vi "AprilTag Target Package Code 1 with integrated camera.vi"(1 "Instance":i32) -> (0 "Camera Name":string="cam0")   [LabVIEW 2025]
uses:
  <vilib>/vision/Image Controls.llb/IMAQ Image.ctl
  <vilib>/Utility/config.llb/NI_LVConfig.lvlib
  Camera Set Up/Event/Event Setup Types.ctl
  State Machine/AprialTag States.ctl
  State Machine/AprialTag Main Cluster.ctl
  Steam Type.ctl
  <vilib>/ptbypt/NI_PtbyPt.lvlib
  <vilib>/Utility/config.llb/Read Key (String).vi
  <vilib>/Utility/config.llb/Write Key (String).vi
  Camera Set Up/Ctrl/White Balance.ctl
  <vilib>/userDefined/High Color/IMAQdx.ctl
  Main State Machine/Ctrl's/Main States.ctl
  Main State Machine/Ctrl's/Main Queue.ctl
  Main State Machine/Ctrl's/Main Cluster.ctl
  <vilib>/vision/driver/NI_Vision_Acquisition_Software.lvlib
  <vilib>/vision/NI_Vision_Development_Module.lvlib
  <resource>/objmgr/imaqdx.rc
  <vilib>/regexp/Match Regular Expression.xnode
  cef373c4-9c7f-4541-9f08-8c9f27cfdef0.vi
  Camera Info.ctl
panel:
  in  "Main":enum32{"Page 1", "Page 2", "Page 3"}(tab)
  out "Target Pitch":dbl[](array[numeric]) caption="Tag Pitch (deg)" format="%.1f"
  out "Target Yaw":dbl[](array[numeric]) caption="Tag Yaw (deg)" format="%.1f"
  out "Tag ID":dbl[](array[numeric]) caption="Tag Number"
  out "Image":T1(plugin-control)
  in  "Settings":bool
  in  "Save":bool
  in  "Tools":bool
  out "FPS":dbl format="%#.0f"
  out "Distance":dbl[](array[numeric]) caption="Tag Distance (in)" format="%.1f"
  out "Angle":dbl[](array[numeric]) caption="Center Angle (deg)" format="%.1f"
  out "Height":i32=360
  out "Width":i32=640
  in  "Home":bool
  in  "Robot Calibration Cluster":T2={"Camera Height on robot (in)"=9.5, "Camera Angle on the robot (deg)"=2.5, "Camera FOV Vert View Angle (deg)"=26.5, "Camera FOV Hor View Angle (deg)"=68.5, "Camera Focal Length (mm)"=10.0, "Target size (in)"=6.5} {"Camera FOV Hor View Angle (deg)" format="%#_13g"; "Camera Focal Length (mm)" format="%#_13g"; "Target size (in)" format="%#_13g"; "Camera FOV Vert View Angle (deg)" format="%#_13g"; "Camera Angle on the robot (deg)" format="%#_13g"; "Camera Height on robot (in)" format="%#_13g"}
  in  "decimate":dbl=4.0 format="%#_13g"
  out "Data to Send":dbl[][](array[numeric])
  out "Greyscale":bool
  out "Height 2":u32=360
  out "Width 2":u32=640
  out "Frames per Second":dbl format="%#.1f"
  in  "Gamma":i32(slide)=50 min=1 max=100 scale=0.0..100.0
  in  "Brightness":i32(slide)=50 min=1 max=100 scale=0.0..100.0
  in  "Exposure":i32(slide)=50 min=1 max=100 scale=0.0..100.0
  in  "Save 2":bool caption="Save"
  in  "Close":bool
  in  "Gain":i32(slide)=50 min=1 max=100 scale=0.0..100.0
  in  "Contrast":i32(slide)=50 min=1 max=100 scale=0.0..100.0
  in  "Sharpness":i32(slide)=50 min=1 max=100 scale=0.0..100.0
  in  "VideoMode":u16(ring)=20 items=["640x480 MJPG 60.00fps", "640x480 YUY2 60.00fps", "1280x720 MJPG 60.00fps", "1280x720 YUY2 60.00fps", "1600x1304 MJPG 60.00fps", "1600x1304 YUY2 60.00fps"]
  in  "White Balance":T3=enum."Hold current"
  out "Camera Name 2":string="cam1"
  out "Camera Image":T1(plugin-control)
  in  "Hue":i32(slide)=50 min=1 max=100 scale=0.0..100.0
  in  "Saturation":i32(slide)=50 min=1 max=100 scale=0.0..100.0
  out "Camera Name 3":string="cam0"
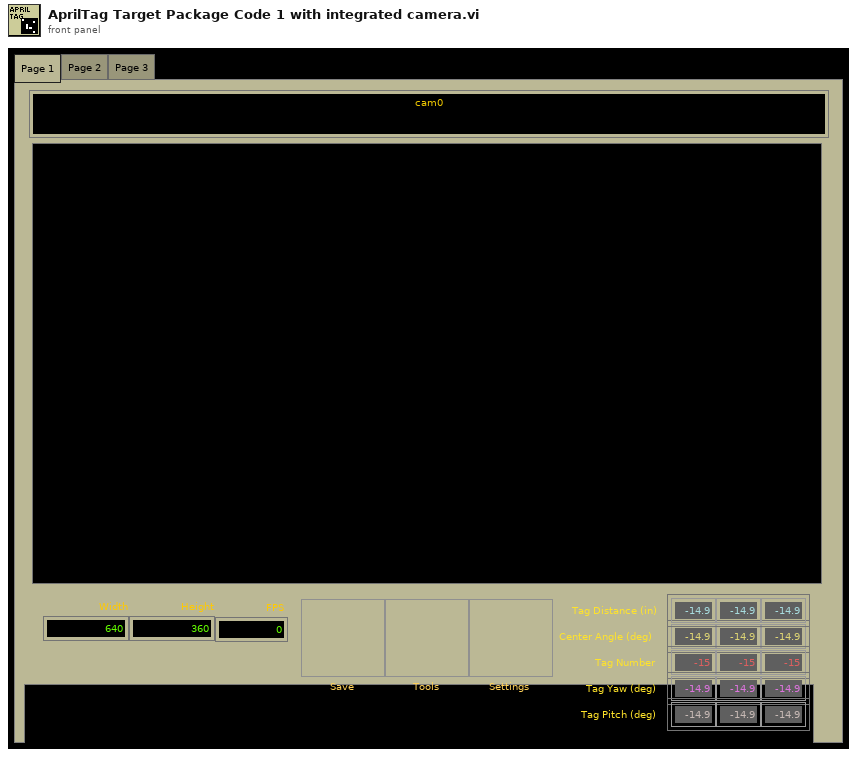
[diagram p1: front panel]
types:
  T1 = typedef "IMAQ Image.ctl" = refnum<image>
  T2 = typedef "Camera Info.ctl" = cluster{"Camera Height on robot (in)":dbl, "Camera Angle on the robot (deg)":dbl, "Camera FOV Vert View Angle (deg)":dbl, "Camera FOV Hor View Angle (deg)":dbl, "Camera Focal Length (mm)":dbl, "Target size (in)":dbl}
  T3 = typedef "White Balance.ctl" = enum16{"Auto", "Fixed indoor", "Fixed outdoor 1", "Fixed outdoor 2", "Fixed fluorescent 1", "Fixed fluorescent 2", "Hold current", "Custom"}
  T4 = typedef "AprialTag Main Cluster.ctl" = cluster{"AprilTage FIFO":T5[], "Camera Name":string, "AprilTag path":path, "Control Ref's":refnum<vi>[], "Main Image":T1, "Timeout":i32, "EDIT Settings":bool, "Calibration path":path, "Camera Number":dbl}
  T5 = typedef "AprialTag States.ctl" = enum16{"Message Dispatcher", "INI", "Open", "Save", "Exit"}
  T6 = typedef "Main Cluster.ctl" = cluster{"Main Queue":T7, "error":errorcluster, "Camera":T9, "Camera Session":T9, "Image In":T1, "White Balance":T3, "Attr String":string[], "Values":u16[], "VideoMode":u16, "Exposure":i32, "Reset":bool, "Greyscale":bool, "Controls":refnum<vi>[], "INI path":path, "INI File Found":bool, "Open And Save Controls":refnum<vi>[]}
  T7 = typedef "Main Queue.ctl" = T8[]
  T8 = typedef "Main States.ctl" = enum16{"Message Dispatcher", "INI", "End Session", "Camera Process Settings", "Get Values", "Get VideoMode", "Open Settings", "Save Settings", "Set Value", "Set VideoMode", "Set WB", "Setup Camera", "Start Session", "Exit"}
  T9 = typedef "IMAQdx.ctl" = refnum<k21>
  T10 = typedef "Event Setup Types.ctl" = enum16{"Default", "Camera Loop Started", "GreyScale", "Reset Team Number", "Save Data", "Exit"}
  T11 = enum32{"Invalid", "Standard", "Closed", "Hidden", "Minimized", "Maximized"}
  T12 = enum32{"Invalid", "Default", "Floating", "Floating/Auto-Hide", "Modal"}
  T13 = typedef "Steam Type.ctl" = enum8{"Unknown", "Apriltag", "Algae", "Coral"}
  T14 = typedef "Event Setup Types.ctl" = enum16{"Default", "Camera Loop Started", "Close Settings", "GreyScale", "Open Front Panel", "Reset Team Number", "Save Data", "Exit"}
  T15 = cluster{"tag ID":i32, "Center":cluster{"X":dbl, "Y":dbl}, "homography matrix":dbl[], "decision margin":dbl, "Hamming Dist":i32, "corner points":cluster{"X":dbl, "Y":dbl}[], "Tag Family":string}[]
  T16 = typedef "AprilTag Target Fields.ctl" = cluster{"diameter points":cluster{"first point":cluster{"x":dbl, "y":dbl}, "projected point":cluster{"x":dbl, "y":dbl}}, "normalized center":cluster{"x":dbl, "y":dbl}, "Overall Score":dbl, "Distance (ft)":dbl, "Offset Angle":dbl, "Tag corner points":cluster{"X":dbl, "Y":dbl}[], "Tag Center":cluster{"X":dbl, "Y":dbl}, "Tag Yaw":dbl, "Tag Pitch":dbl, "Target Roll (deg)":dbl, "AprilTag Number":i32, "homography matrix":dbl[]}
  T17 = typedef "Image Type" = u32
  T18 = typedef "NI_LVConfig.lvlib/Config Data RefNum.ctl" = refnum<k1>
  T19 = cluster{"Video Mode":u32, "Video Mode Name":string}[]
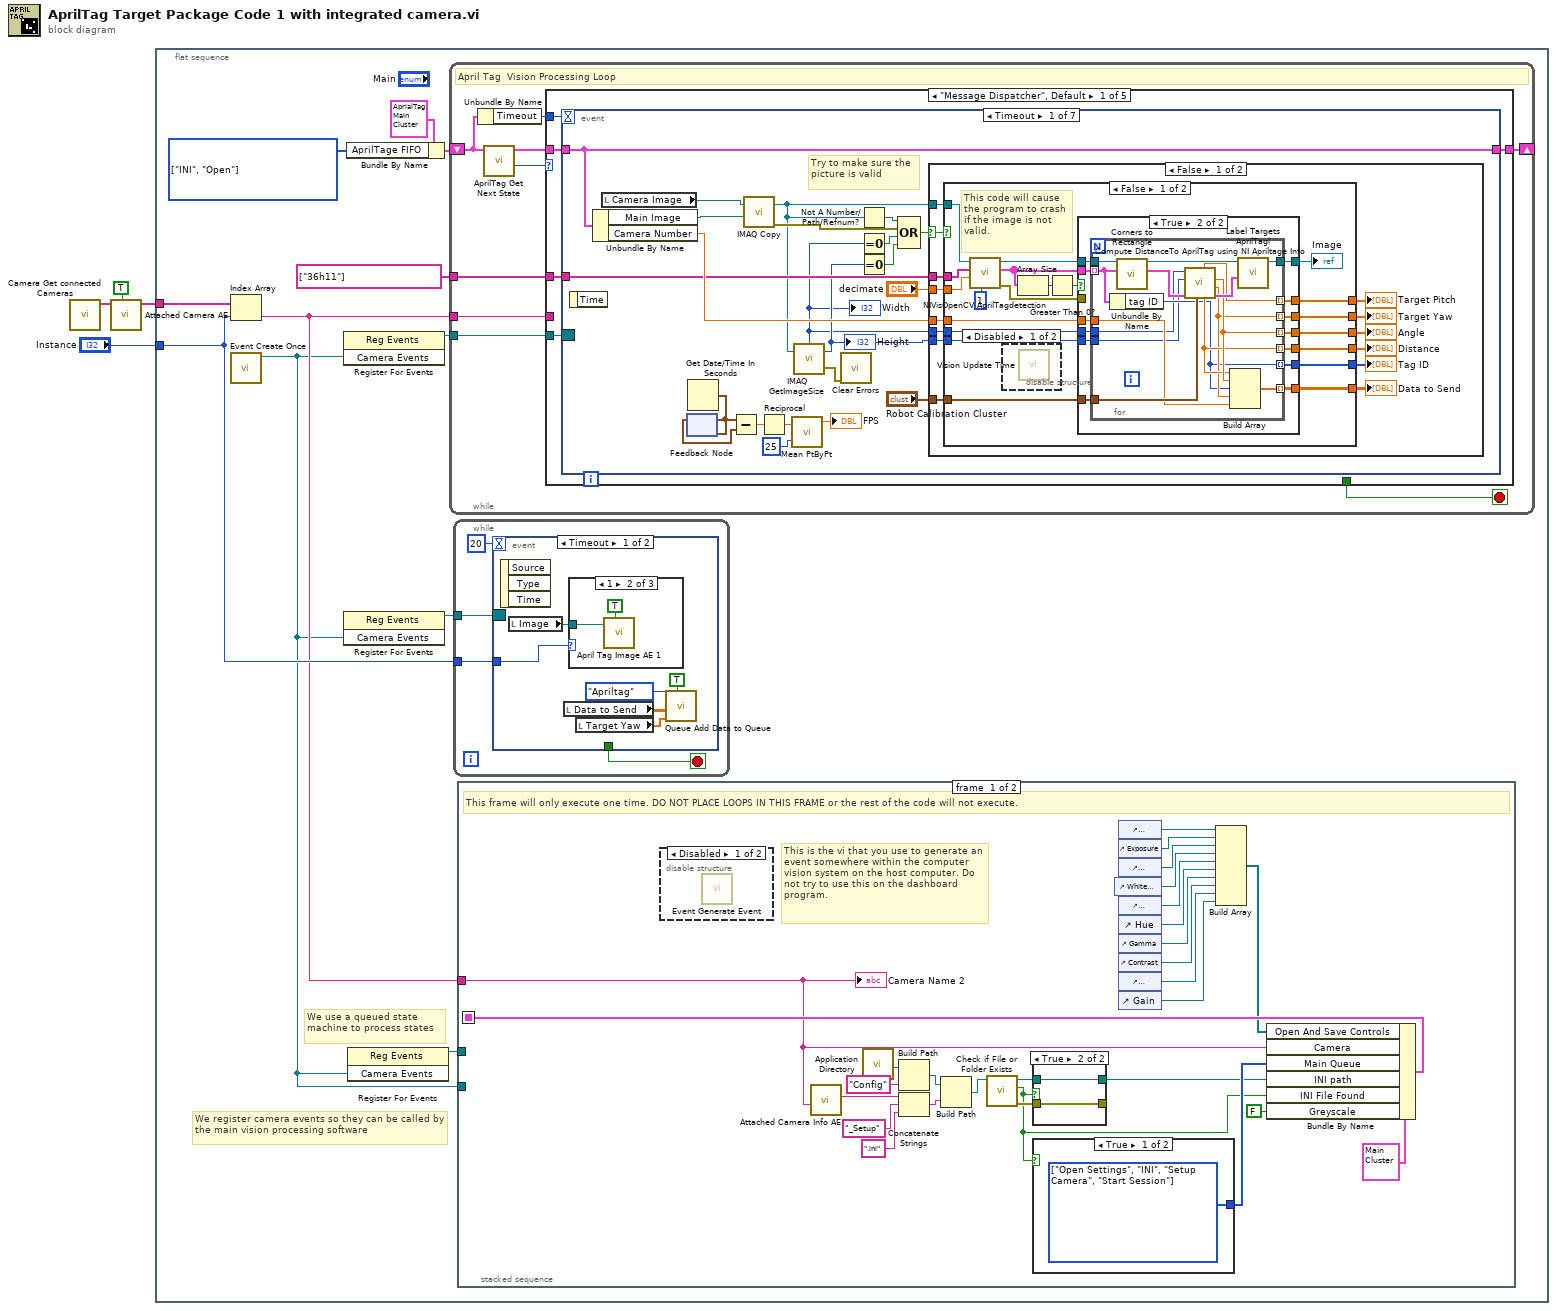
[diagram p0: block diagram]
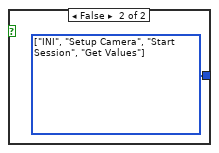
[diagram p2: hidden frame]
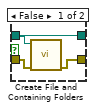
[diagram p3: hidden frame]
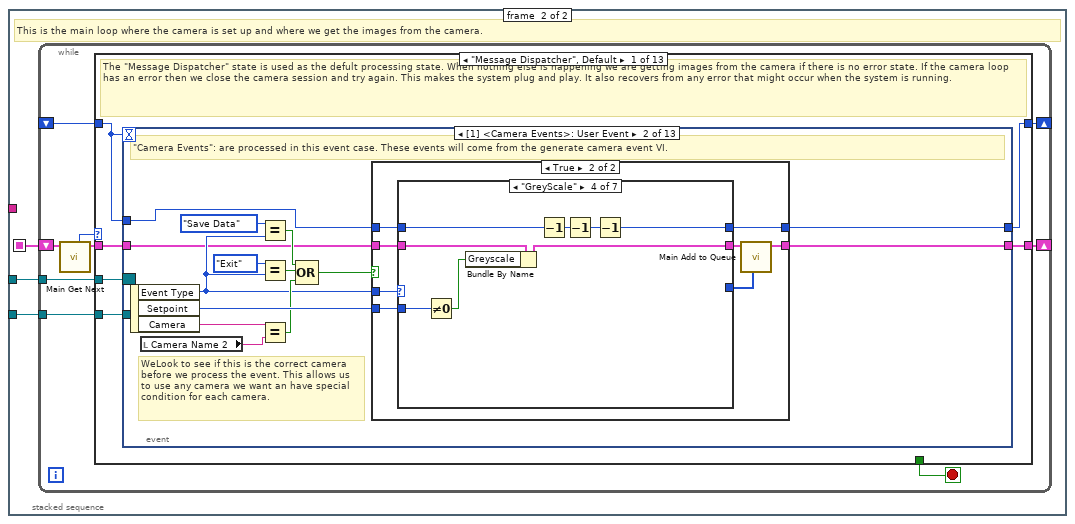
[diagram p5: hidden frame]
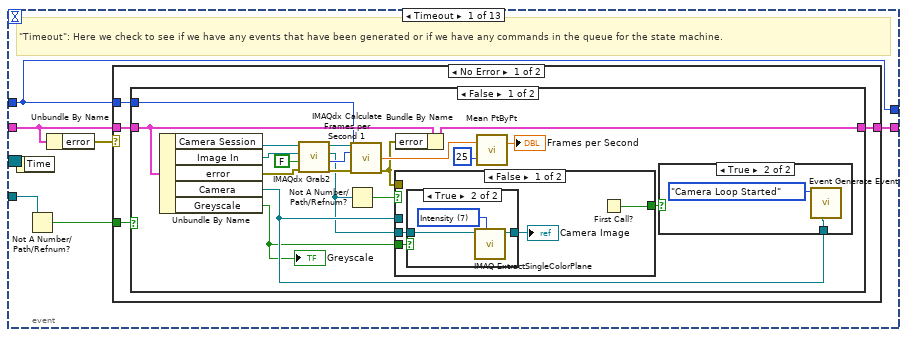
[diagram p6: hidden frame]
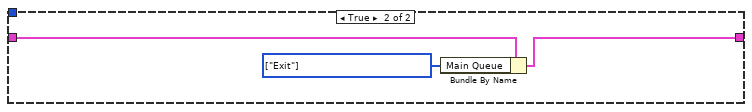
[diagram p10: hidden frame]
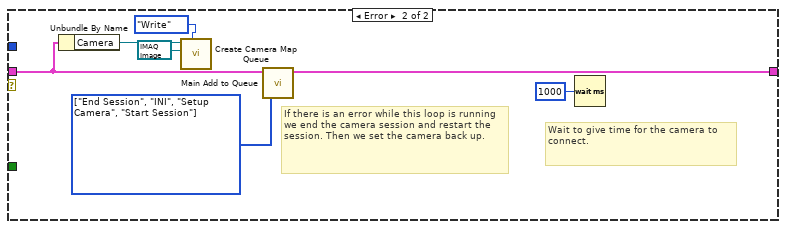
[diagram p11: hidden frame]
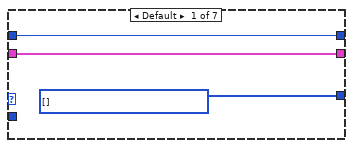
[diagram p13: hidden frame]
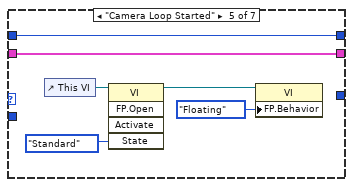
[diagram p16: hidden frame]
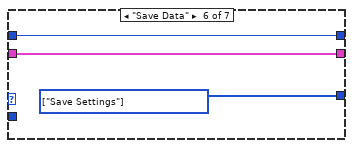
[diagram p17: hidden frame]
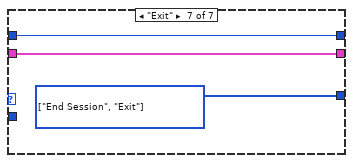
[diagram p18: hidden frame]
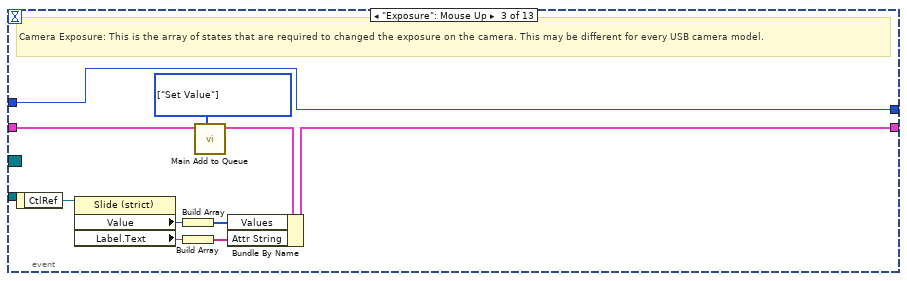
[diagram p19: hidden frame]
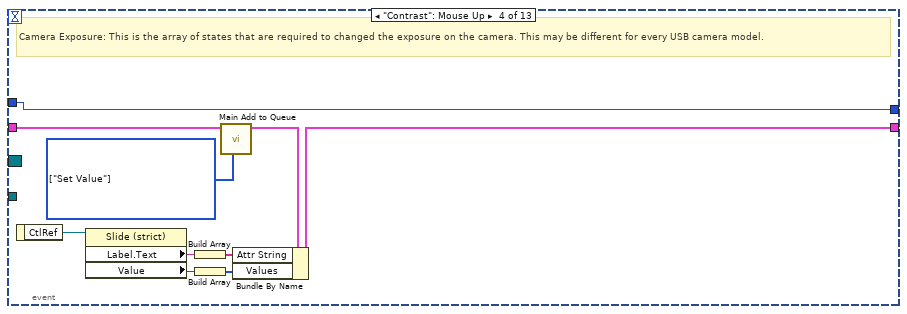
[diagram p20: hidden frame]
diagram:
  n1 = call "Camera Get connected Cameras.vi"() -> ("Camera List"=w4:string[])  [unwired: 10 in, 1 out]
  n2 = call "Attached Camera AE.vi"("Update"=TRUE, "Camera List in"=w4) -> ("Camera List out"=w2:string[])  [unwired: 9 in]
  n3 = flat-sequence {
    tunnel: w2 -> [w8]
    tunnel: "Instance" -> [w7]
    frame #0 {
      w12 = T5[] [enum."INI", enum."Open"] items=["Message Dispatcher", "INI", "Open", "Save", "Exit"] ("AprilTage FIFO")
      # "We register camera events so they can be called by the main vision processing software"
      # "We use a queued state machine to process states"
      n4 = Index Array(array=w8, index=w7) -> (element=w6:string)
      n5 = call "Event Create Once.vi"() -> ("Camera Events"=w5:refnum<user-event>)  [unwired: 10 in, 1 out]
      n6 = register-events(w5) -> (reference out=w15:refnum<event-registration>)  [unwired: 2 in, 1 out]
      n7 = register-events(w5) -> (reference out=w10:refnum<event-registration>)  [unwired: 2 in, 1 out]
      n8 = Bundle By Name(cluster=T4 {"AprilTage FIFO"=[], "Camera Name"="", "AprilTag path"=path "", "Control Ref's"=[], "Main Image"=refnum, "Timeout"=5, "EDIT Settings"=FALSE, "Calibration path"=path "", "Camera Number"=0.0} ("AprilTag Main Cluster out"), "AprilTage FIFO"=w12) -> (w13:T4)
      n9 = register-events(w5) -> (reference out=w9:refnum<event-registration>)  [unwired: 2 in, 1 out]
      n10 = while {
        tunnel: w15 -> [w762]
        shift-right: [w758] -> _
        shift-left: w13 -> [w756]
        tunnel: string[] ["36h11"] ("Tag Familys") -> [w755]
        tunnel: w6 -> [w754]
        stop <- w761 stop-if-true
        # "April Tag  Vision Processing Loop"
        n11 = Unbundle By Name(w756) -> ("Timeout"=w757:i32)
        n12 = call "AprilTag Get Next State.vi"("AprilTag Main Cluster in"=w756) -> ("Next State"=w759:T5, "AprilTag Main Cluster out"=w760:T4)  [unwired: 9 in]
        n13 = case shown="\"Message Dispatcher\", Default" w759 {
          tunnel: w762 -> [w767 _ _ _ _]
          tunnel: [_ _ _ _ TRUE] -> w761
          tunnel: w760 -> [w765 w914 w931 w968 w984]
          tunnel: [w766 w913 w930 w968 w984] -> w758
          tunnel: w757 -> [w764 _ _ _ _]
          tunnel: w755 -> [w763 _ _ _ _]
          tunnel: w754 -> [_ w890 w920 _ _]
          frame "Message Dispatcher", Default {
            n14 = event shown="[0] Timeout" {
              selector: w767 -> [_ _ _ _ _ _ _]
              dyn-events: _ -> [_ _ _ _ _ _ _]
              timeout: w764 -> [_ _ _ _ _ _ _]
              tunnel: w765 -> [w789 w856 w879 w880 w882 w886 w888]
              tunnel: [w789 w858 w878 w880 w882 w885 w888] -> w766
              tunnel: w763 -> [w785 _ _ _ _ _ _]
              event Timeout {
                # "Try to make sure the picture is valid"
                n15 = event-data() -> ()  [unwired: 1 in, 1 out]
                n16 = Unbundle By Name(w789) -> ("Main Image"=w784:T1, "Camera Number"=w787:dbl)
                n17 = local read "Camera Image"() -> (w768:T1)
                n18 = Get Date/Time In Seconds() -> (seconds since 1Jan1904=w773:timestamp)
                n19 = feedback #1(w773) -> (w774:timestamp)
                n20 = feedback-in #1(w773) -> ()
                n21 = Subtract(x=w773, y=w774) -> (x-y=w771:dbl)
                n22 = call "IMAQ Copy"("Image Dst"=w784, "Image Src"=w768) -> ("error out"=w783:errorcluster, "Image Dst Out"=w776:T1)  [unwired: 4 in]
                n23 = Reciprocal(x=w771) -> (1/x=w772:dbl)
                n24 = call <vilib>:"Mean PtByPt.vi"("x"=w772, "sample length"=25) -> ("mean"=→"FPS":dbl)  [unwired: 2 in, 1 out]
                n25 = call "IMAQ GetImageSize"("Image"=w776) -> ("Y Resolution"=w778:i32, "X Resolution"=w777:i32, "error out"=w775:errorcluster)  [unwired: 3 in]
                "Height" <- w778
                "Width" <- w777
                n26 = call <vilib>:"Clear Errors.vi"("error in (no error)"=w775) -> ()  [unwired: 5 in, 2 out]
                n27 = Not A Number/Path/Refnum?(number/path/refnum=w776) -> (NaN/Path/Refnum?=w782:bool)
                n28 = Equal To 0?(x=w777) -> (x = 0?=w780:bool)
                n29 = Equal To 0?(x=w778) -> (x = 0?=w779:bool)
                n30 = Compound Arithmetic op=OR(w782, w783, w780, w779) -> (w781:bool)
                n31 = case shown="False" w781 {
                  selector: w781 -> [w794 _]
                  tunnel: w785 -> [w803 _]
                  tunnel: "Robot Calibration Cluster" -> [w802 _]
                  tunnel: w787 -> [w797 _]
                  tunnel: w776 -> [w796 _]
                  tunnel: "decimate" -> [w795 _]
                  tunnel: w778 -> [w792 _]
                  tunnel: w777 -> [w791 _]
                  frame False {
                    n32 = case shown="False" w794 {
                      tunnel: w803 -> [w823 _]
                      tunnel: w802 -> [w822 _]
                      tunnel: [w817 _] -> w790
                      tunnel: [w816 _] -> w801
                      tunnel: [w815 _] -> w793
                      tunnel: [w814 _] -> w800
                      tunnel: [w813 _] -> w799
                      tunnel: [w812 _] -> w798
                      tunnel: w797 -> [w811 _]
                      tunnel: w796 -> [w808 _]
                      tunnel: w795 -> [w809 _]
                      tunnel: w792 -> [w805 _]
                      tunnel: w791 -> [w804 _]
                      frame False {
                        # "This code will cause the program to crash if the image is not valid."
                        n33 = call "NIVisOpenCV AprilTagdetection.vi"("threads"=1, "decimate"=w809, "Tag Familys"=w823, "Image Src"=w808) -> ("error out"=w818:errorcluster, "Detected Tags"=w821:T15, "Image Dst Out"=w807:T1)  [unwired: 4 in, 1 out]
                        n34 = disable-structure shown="Disabled" {
                          frame Disabled {
                            n35 = call "Vision Update Time.vi"() -> ()  [unwired: 12 in]
                          }
                          frame Enabled {
                          }
                        }
                        n36 = Array Size(array=w821) -> (size(s)=w820:i32)
                        n37 = Greater Than 0?(x=w820) -> (x > 0?=w819:bool)
                        n38 = case shown="True" w819 {
                          tunnel: w807 -> [w824 w837]
                          tunnel: w821 -> [_ w836]
                          tunnel: [w824 w827] -> w810
                          tunnel: w818 -> [_ _]
                          tunnel: w822 -> [_ w835]
                          tunnel: [_ w834] -> w817
                          tunnel: [_ w833] -> w816
                          tunnel: [_ w832] -> w815
                          tunnel: [_ w831] -> w814
                          tunnel: [_ w830] -> w813
                          tunnel: [_ w829] -> w812
                          tunnel: w811 -> [_ w828]
                          tunnel: w805 -> [_ w826]
                          tunnel: w804 -> [_ w825]
                          frame False {
                          }
                          frame True {
                            n39 = for {
                              tunnel: w836 -> [w851] mode=indexing
                              tunnel: w837 -> [w840]
                              tunnel: [w852] -> w827
                              tunnel: [w841] -> w831 mode=indexing
                              tunnel: [w846] -> w829 mode=indexing
                              tunnel: [w848] -> w830 mode=indexing
                              tunnel: w835 -> [w847]
                              tunnel: [w845] -> w832 mode=indexing
                              tunnel: [w844] -> w834 mode=indexing
                              tunnel: [w843] -> w833 mode=indexing
                              tunnel: w828 -> [w842]
                              tunnel: w826 -> [w839]
                              tunnel: w825 -> [w838]
                              n40 = Unbundle By Name(w851) -> ("tag ID"=w841:i32)
                              n41 = call "Corners to Rectangle.vi"("tag info"=w851) -> ("output cluster"=w850:T16)  [unwired: 10 in]
                              n42 = call "Compute DistanceTo AprilTag using NI Apriltage Info.vi"("Robot Calibration Cluster"=w847, "results"=w850, "Y Resolution"=w839, "X Resolution"=w838) -> ("results out"=w849:T16, "Target Yaw (deg)"=w845:dbl, "Offset Angle"=w848:dbl, "Distance from target (in)"=w846:dbl, "Target Pitch (deg)"=w843:dbl)  [unwired: 2 in, 1 out]
                              n43 = Build Array(w846, w848, w841, w845, w842) -> (w844:dbl[])
                              n44 = call "Label Targets AprilTagl.vi"("results"=w849, "Image in"=w840) -> ("Image out"=w852:T1)  [unwired: 9 in]
                            }
                          }
                        }
                        "Image" <- w810
                      }
                      frame True {
                      }
                    }
                    "Distance" <- w798
                    "Angle" <- w799
                    "Tag ID" <- w800
                    "Target Yaw" <- w793
                    "Target Pitch" <- w801
                    "Data to Send" <- w790
                  }
                  frame True {
                  }
                }
              }
              event User Event {
                n45 = event-data() -> ("Camera"=w854:string, "Event Type"=w857:T10)  [unwired: 1 in]
                n46 = Unbundle By Name(w856) -> ("Camera Name"=w855:string)
                n47 = Equal?(x=w855, y=w854) -> (x = y?=w853:bool)
                n48 = case shown="\"Save Data\"" w857 {
                  tunnel: w856 -> [w859 w861 w866 w867 w868 w869 w872 w875]
                  tunnel: [w859 w865 w866 w867 w868 w869 w871 w874] -> w858
                  tunnel: w853 -> [_ _ _ _ _ _ _ _]
                  frame "Default" {
                  }
                  frame "Camera Loop Started" {
                    n49 = Unbundle By Name(w861) -> ("Camera Name"=w860:string)
                    n50 = call "Event Generate Event.vi"("Camera Name"=w860, "Setpoint"=i64 1, "Event Type"=Event_Setup_Types."GreyScale") -> ()  [unwired: 9 in]
                    n51 = Bundle By Name(cluster=w861, "Timeout"=10) -> (w865:T4)
                  }
                  frame "Default" {
                  }
                  frame "GreyScale" {
                  }
                  frame "Camera Loop Started" {
                  }
                  frame "Reset Team Number" {
                  }
                  frame "Save Data" {
                    w870 = T5[] [enum."Save"] items=["Message Dispatcher", "INI", "Open", "Save", "Exit"] ("AprilTage FIFO")
                    n52 = Bundle By Name(cluster=w872, "AprilTage FIFO"=w870) -> (w871:T4)
                  }
                  frame "Exit" {
                    w873 = T5[] [enum."Exit"] items=["Message Dispatcher", "INI", "Open", "Save", "Exit"] ("AprilTage FIFO")
                    n53 = Bundle By Name(cluster=w875, "AprilTage FIFO"=w873) -> (w874:T4)
                  }
                }
              }
              event "Camera Name": Value Change {
                w877 = T5[] [enum."INI", enum."Save"] items=["Message Dispatcher", "INI", "Open", "Save", "Exit"] ("AprilTage FIFO")
                n54 = event-data() -> ("NewVal"=w876:string)  [unwired: 1 in]
                n55 = Bundle By Name(cluster=w879, "Camera Name"=w876, "AprilTage FIFO"=w877) -> (w878:T4)
              }
              event "Tools": Mouse Up {
                n56 = event-data() -> ()  [unwired: 1 in, 1 out]
                n57 = property on="Main" class="TabCtl (strict)"("Value"=enum32{"Page 1", "Page 2"}."Page 2" ("Main")) -> ()  [unwired: 2 in, 2 out]
              }
              event "Home": Mouse Up {
                n58 = event-data() -> ()  [unwired: 1 in, 1 out]
                n59 = property on="Main" class="TabCtl (strict)"("Value"=enum32{"Page 1", "Page 2"}."Page 1" ("Main")) -> ()  [unwired: 2 in, 2 out]
              }
              event "Save": Mouse Up {
                w884 = T5[] [enum."Save"] items=["Message Dispatcher", "INI", "Open", "Save", "Exit"] ("AprilTage FIFO")
                n60 = event-data() -> ()  [unwired: 1 in, 1 out]
                n61 = Bundle By Name(cluster=w886, "AprilTage FIFO"=w884) -> (w885:T4)
              }
              event "Settings": Mouse Up {
                n62 = event-data() -> ()  [unwired: 1 in, 1 out]
                n63 = Unbundle By Name(w888) -> ("Camera Name"=w887:string)
                n64 = call "Event Generate Event.vi"("Camera Name"=w887, "Event Type"=Event_Setup_Types."Open Front Panel") -> ()  [unwired: 10 in]
              }
            }
          }
          frame "INI" {
            w911 = T17 0 items=["Grayscale (U8)", "Grayscale (I16)", "Grayscale (SGL)", "Complex (CSG)", "RGB (U32)", "HSL (U32)", "RGB (U64)", "Grayscale (U16)"] ("Image Type")
            n65 = call <vilib>:"Application Directory.vi"() -> ("Application Directory"=w904:path)
            n66 = Build Path(base path=w904, name or relative path="Config") -> (appended path=w902:path)
            n67 = Concatenate Strings(w890, ".png" ("name or relative path")) -> (w906:string)
            n68 = call "Event Generate Event.vi"("Camera Name"=w890, "Setpoint"=i64 0, "Event Type"=Event_Setup_Types."GreyScale") -> ()  [unwired: 9 in]
            n69 = Build Path(base path=w902, name or relative path=w906) -> (appended path=w901:path)
            n70 = call <vilib>:"Check if File or Folder Exists.vi"("error in (no error)"=errorcluster {"status"=FALSE, "code"=0, "source"=""}, "path"=w901) -> ("error out"=w898:errorcluster, "file or folder exists?"=w899:bool, "dup path"=w900:path)  [unwired: 7 in]
            n71 = case shown="True" w899 {
              tunnel: [w917 w918] -> _
              tunnel: w900 -> [w916 w919]
              tunnel: [w916 w919] -> w896
              tunnel: w898 -> [w915 w918]
              frame False {
                n72 = call <vilib>:"Create File and Containing Folders.vi"("error in (no error)"=w915, "file path"=w916) -> ("error out"=w917:errorcluster)  [unwired: 8 in, 1 out]
              }
              frame True {
              }
            }
            n73 = Concatenate Strings(w890, "AprilTag Main" ("string")) -> (w910:string)
            n74 = Match Pattern(string=w890, regular expression="[1-9]") -> (match substring=w892:string)  [unwired: 1 in, 3 out]
            n75 = call "IMAQ Create"("Image Name"=w910, "Image Type"=w911) -> ("New Image"=w908:T1)  [unwired: 2 in, 2 out]
            n76 = Fract/Exp String To Number(string=w892) -> (number=w891:dbl)  [unwired: 3 in, 1 out]
            n77 = Bundle By Name(cluster=w914, "Camera Name"=w890, "Timeout"=100, "Main Image"=w908, "EDIT Settings"=FALSE, "Calibration path"=w896, "Camera Number"=w891) -> (w913:T4)
            "Camera Name" <- w890
            "Camera Name 3" <- w890
          }
          frame "Open" {
            n78 = call <vilib>:"Application Directory.vi"() -> ("Application Directory"=w934:path)
            n79 = Concatenate Strings(w920, ".ini" ("name or relative path")) -> (w943:string)
            n80 = Build Path(base path=w934, name or relative path="Config") -> (appended path=w932:path)
            n81 = Build Path(base path=w932, name or relative path=w943) -> (appended path=w926:path)
            n82 = call <vilib>:"Check if File or Folder Exists.vi"("error in (no error)"=errorcluster {"status"=FALSE, "code"=0, "source"=""}, "path"=w926) -> ("error out"=w922:errorcluster, "file or folder exists?"=w924:bool, "dup path"=w925:path)  [unwired: 7 in]
            n83 = control-ref of="Main"() -> (w938:refnum<vi>)
            n84 = control-ref of="Robot Calibration Cluster"() -> (w937:refnum<vi>)
            n85 = control-ref of="Camera Name"() -> ()  [unwired: 1 out]
            n86 = case shown="False" w924 {
              tunnel: [w946 w947] -> w935
              tunnel: w925 -> [w945 w948]
              tunnel: [w945 w948] -> w923
              tunnel: w922 -> [w944 w947]
              frame False {
                n87 = call <vilib>:"Create File and Containing Folders.vi"("error in (no error)"=w944, "file path"=w945) -> ("error out"=w946:errorcluster)  [unwired: 8 in, 1 out]
              }
              frame True {
              }
            }
            n88 = Build Array(w938, w937) -> (w929:refnum<vi>[])
            n89 = call <vilib>:"Open Config Data.vi"("error in (no error)"=w935, "configuration file path"=w923) -> ("error out"=w939:errorcluster, "refnum"=w942:T18)  [unwired: 7 in, 1 out]
            n90 = for {
              tunnel: "Info" ("Camera Name") -> [w961]
              tunnel: w929 -> [w959] mode=indexing
              shift-right: [w963] -> w941
              shift-left: w942 -> [w964]
              shift-right: [w962] -> w940
              shift-left: w939 -> [w960]
              tunnel: [w954] -> _ mode=indexing
              tunnel: errorcluster {"status"=FALSE, "code"=0, "source"=""} ("error out") -> [w953]
              tunnel: [w949] -> _ mode=indexing
              n91 = property class="Ctl"(reference=w959, error in=w953) -> (reference out=w957:refnum<vi>, error out=w955:errorcluster, "Label.Text"=w958:string, "Value"=w951:variant)
              n92 = Variant To Flattened String(Variant=w951) -> (1:w950:i16[])  [unwired: 1 out]
              n93 = call-poly <vilib>:"Read Key.vi"("section"=w961, "error in (no error)"=w960, "key"=w958, "refnum"=w964) -> ("error out"=w962:errorcluster, "value"=w956:string, "refnum out"=w963:T18)  [unwired: 4 in, 1 out]
              n94 = Flattened String To Variant(6:w956, 7:w950) -> (0:w949:errorcluster, 3:w952:variant)  [unwired: 1 in]
              n95 = property class="Ctl"(reference=w957, error in=w955, "Value"=w952) -> (error out=w954:errorcluster)  [unwired: 1 out]
            }
            n96 = call <vilib>:"Close Config Data.vi"("error in (no error)"=w940, "refnum"=w941) -> ()  [unwired: 8 in, 2 out]
            n97 = Bundle By Name(cluster=w931, "Control Ref's"=w929, "AprilTag path"=w923) -> (w930:T4)
          }
          frame "Save" {
            n98 = Unbundle By Name(w968) -> ("Control Ref's"=w966:refnum<vi>[], "AprilTag path"=w967:path)
            n99 = call <vilib>:"Open Config Data.vi"("configuration file path"=w967) -> ("error out"=w969:errorcluster, "refnum"=w972:T18)  [unwired: 8 in, 1 out]
            n100 = for {
              tunnel: "Info" ("Camera Name") -> [w978]
              shift-right: [w981] -> w971
              shift-left: w972 -> [w982]
              shift-right: [w980] -> w970
              shift-left: w969 -> [w979]
              tunnel: w966 -> [w973] mode=indexing
              n101 = property class="Ctl"(reference=w973, error in=w979) -> (error out=w975:errorcluster, "Label.Text"=w977:string, "Value"=w976:variant)  [unwired: 1 out]
              n102 = Variant To Flattened String(Variant=w976) -> (data string=w974:string)  [unwired: 1 out]
              n103 = call-poly <vilib>:"Write Key.vi"("section"=w978, "error in (no error)"=w975, "value"=w974, "key"=w977, "refnum"=w982) -> ("error out"=w980:errorcluster, "refnum out"=w981:T18)  [unwired: 4 in, 1 out]
            }
            n104 = call <vilib>:"Close Config Data.vi"("error in (no error)"=w970, "refnum"=w971) -> ()  [unwired: 8 in, 2 out]
          }
          frame "Exit" {
            n105 = Unbundle By Name(w984) -> ("Main Image"=w983:T1)
            n106 = call "IMAQ Dispose"("Image"=w983) -> ()  [unwired: 5 in, 1 out]
          }
        }
      }
      n107 = while {
        tunnel: w10 -> [w740]
        tunnel: w7 -> [w737]
        stop <- w738 stop-if-true
        n108 = event shown="[0] Timeout" {
          selector: w740 -> [_ _]
          dyn-events: _ -> [_ _]
          timeout: 20 -> [_ _]
          tunnel: [_ w751] -> w738
          tunnel: w737 -> [w745 _]
          event Timeout {
            n109 = event-data() -> ()  [unwired: 1 in, 3 out]
            n110 = local read "Image"() -> (w746:T1)
            n111 = local read "Data to Send"() -> (w742:dbl[][])
            n112 = case shown="1" w745 {
              tunnel: w746 -> [_ w747 w750]
              frame 0, Default {
              }
              frame 1 {
                n113 = call "April Tag Image AE 1.vi"("Update"=TRUE, "Apriltag Image in"=w747) -> ()  [unwired: 9 in, 1 out]
              }
              frame 2 {
                n114 = call "April Tag Image AE 2.vi"("Update"=TRUE, "Apriltag Image in"=w750) -> ()  [unwired: 9 in, 1 out]
              }
            }
            n115 = local read "Target Yaw"() -> (w741:dbl[])
            n116 = call "Queue Add Data to Queue.vi"(7:TRUE ("Update"), "yaw"=w741, "Info in"=w742, "Stream Type"=Steam_Type."Apriltag") -> ()  [unwired: 8 in]
          }
          event User Event {
            n117 = event-data() -> ("Event Type"=w752:T10)  [unwired: 1 in, 1 out]
            n118 = case shown="\"Exit\"" w752 {
              tunnel: [_ TRUE] -> w751
              frame Default {
              }
              frame "Exit" {
              }
            }
          }
        }
      }
      n119 = stacked-sequence {
        seq-local: [w36 _] -> [_ w53]
        tunnel: w9 -> [_ w52]
        tunnel: w5 -> [_ w51]
        tunnel: w6 -> [w16 _]
        frame #0 {
          # "This is the vi that you use to generate an event somewhere within the computer vision system on the host computer. Do not try to use this on the dashboard program."
          # "This frame will only execute one time. DO NOT PLACE LOOPS IN THIS FRAME or the rest of the code will not execute."
          n120 = disable-structure shown="Disabled" {
            frame Disabled {
              n121 = call "Event Generate Event.vi"() -> ()  [unwired: 12 in]
            }
            frame Enabled {
            }
          }
          n122 = call "Attached Camera Info AE.vi"("InterfaceName"=w16) -> ("Serial Number"=w19:string)  [unwired: 10 in]
          n123 = call <vilib>:"Application Directory.vi"() -> ("Application Directory"=w41:path)
          n124 = Build Path(base path=w41, name or relative path="Config") -> (appended path=w34:path)
          n125 = Concatenate Strings(w19, "_Setup" ("string"), ".ini" ("name or relative path")) -> (w42:string)
          n126 = Build Path(base path=w34, name or relative path=w42) -> (appended path=w32:path)
          n127 = call <vilib>:"Check if File or Folder Exists.vi"("path"=w32) -> ("error out"=w33:errorcluster, "file or folder exists?"=w21:bool, "dup path"=w31:path)  [unwired: 8 in]
          n128 = case shown="True" w21 {
            tunnel: [w48 w49] -> _
            tunnel: w33 -> [w47 w49]
            tunnel: w31 -> [w46 w50]
            tunnel: [w46 w50] -> w22
            frame False {
              n129 = call <vilib>:"Create File and Containing Folders.vi"("error in (no error)"=w47, "file path"=w46) -> ("error out"=w48:errorcluster)  [unwired: 8 in, 1 out]
            }
            frame True {
            }
          }
          n130 = case shown="True" w21 {
            tunnel: [w44 w45] -> w35
            frame True {
              w44 = T7 [enum."Open Settings", enum."INI", enum."Setup Camera", enum."Start Session"] items=["Message Dispatcher", "INI", "End Session", "Camera Process Settings", "Get Values", "Get VideoMode", "Open Settings", "Save Settings", "Set Value", "Set VideoMode", "Set WB", "Setup Camera", "Start Session", "Exit"] ("Main Queue")
            }
            frame False {
              w45 = T7 [enum."INI", enum."Setup Camera", enum."Start Session", enum."Get Values"] items=["Message Dispatcher", "INI", "End Session", "Camera Process Settings", "Get Values", "Get VideoMode", "Open Settings", "Save Settings", "Set Value", "Set VideoMode", "Set WB", "Setup Camera", "Start Session", "Exit"] ("Main Queue")
            }
          }
          n131 = control-ref of="White Balance"() -> (w29:refnum<vi>)
          n132 = control-ref of="Brightness"() -> (w37:refnum<vi>)
          n133 = control-ref of="Exposure"() -> (w38:refnum<vi>)
          n134 = control-ref of="VideoMode"() -> (w30:refnum<vi>)
          n135 = control-ref of="Saturation"() -> (w28:refnum<vi>)
          n136 = control-ref of="Hue"() -> (w27:refnum<vi>)
          n137 = control-ref of="Gamma"() -> (w26:refnum<vi>)
          n138 = control-ref of="Contrast"() -> (w25:refnum<vi>)
          n139 = control-ref of="Sharpness"() -> (w24:refnum<vi>)
          n140 = control-ref of="Gain"() -> (w23:refnum<vi>)
          n141 = Build Array(w37, w38, w30, w29, w28, w27, w26, w25, w24, w23) -> (w20:refnum<vi>[])
          n142 = Bundle By Name(cluster=T6 {"Main Queue"=[], "error"={"status"=FALSE, "code"=0, "source"=""}, "Camera"="", "Camera Session"="", "Image In"=refnum, "White Balance"=enum."Hold current", "Attr String"=[], "Values"=[], "VideoMode"=0, "Exposure"=50, "Reset"=FALSE, "Greyscale"=FALSE, "Controls"=[], "INI path"=path "", "INI File Found"=FALSE, "Open And Save Controls"=[]} ("Main Cluster Out"), "Open And Save Controls"=w20, "Camera"=w16, "Main Queue"=w35, "INI path"=w22, "INI File Found"=w21, "Greyscale"=FALSE) -> (w36:T6)
          "Camera Name 2" <- w16
        }
        frame #1 {
          # "This is the main loop where the camera is set up and where we get the images from the camera."
          n143 = while {
            shift-right: [w58] -> _
            shift-left: w53 -> [w60]
            tunnel: w52 -> [w57]
            shift-right: [w56] -> _
            shift-left: _ -> [w55]
            tunnel: w51 -> [w54]
            stop <- w62 stop-if-true
            n144 = call "Main Get Next.vi"("Main Cluster In"=w60) -> ("Main Cluster Out"=w59:T6, "Next State"=w61:T8)  [unwired: 9 in]
            n145 = case shown="\"Message Dispatcher\", Default" w61 {
              tunnel: [_ _ _ _ _ _ _ _ _ _ _ _ TRUE] -> w62
              tunnel: w59 -> [w67 w273 w284 w288 w292 w329 w455 w493 w511 w529 w589 w727 w736]
              tunnel: [w68 w268 w281 w286 w291 w328 w452 w493 w510 w539 w584 w721 w736] -> w58
              tunnel: w57 -> [w66 _ _ _ _ _ _ _ _ _ _ _ _]
              tunnel: w55 -> [w64 w274 w282 w287 w298 _ w459 w498 w517 w528 _ w724 w734]
              tunnel: [w63 w274 w282 w287 w298 w307 w459 w498 w517 w528 w567 w724 w734] -> w56
              tunnel: w54 -> [w65 _ _ _ _ _ _ _ _ _ _ _ _]
              frame "Message Dispatcher", Default {
                # "The \"Message Dispatcher\" state is used as the defult processing state. When nothing else is happening we are getting images from the camera if there is no error state. If the camera loop has an error then we close the camera session and try again. This makes the system plug and play. It also recovers from any error that might occur when the system is running."
                n146 = event shown="[1] <Camera Events>: User Event" {
                  selector: w66 -> [_ _ _ _ _ _ _ _ _ _ _ _ _]
                  dyn-events: _ -> [_ _ _ _ _ _ _ _ _ _ _ _ _]
                  timeout: w64 -> [_ _ _ _ _ _ _ _ _ _ _ _ _]
                  tunnel: [w74 w131 w175 w185 w195 w202 w209 w219 w229 w239 w245 w252 w257] -> w68
                  tunnel: w67 -> [w73 w121 w177 w187 w197 w201 w211 w221 w231 w241 w247 w254 w257]
                  tunnel: w65 -> [w71 _ _ _ _ _ _ _ _ _ _ _ _]
                  tunnel: w64 -> [w69 w119 w169 w179 w189 w199 w203 w213 w223 w233 w243 w249 w255]
                  tunnel: [w69 w118 w169 w179 w189 w199 w203 w213 w223 w233 w243 w249 w255] -> w63
                  event Timeout {
                    # "\"Timeout\": Here we check to see if we have any events that have been generated or if we have any commands in the queue for the state machine."
                    n147 = event-data() -> ()  [unwired: 1 in, 1 out]
                    n148 = Not A Number/Path/Refnum?(number/path/refnum=w71) -> (NaN/Path/Refnum?=w70:bool)
                    n149 = Unbundle By Name(w73) -> ("error"=w72:errorcluster)
                    n150 = case shown="No Error" w72 {
                      tunnel: w73 -> [w78 w113]
                      tunnel: [w77 w117] -> w74
                      tunnel: w70 -> [w76 _]
                      tunnel: w69 -> [w75 _]
                      frame No Error {
                        n151 = case shown="False" w76 {
                          tunnel: w78 -> [w97 w110]
                          tunnel: [w86 w109] -> w77
                          tunnel: w75 -> [w82 _]
                          frame False {
                            n152 = Unbundle By Name(w97) -> ("Camera Session"=w96:T9, "Image In"=w95:T1, "error"=w94:errorcluster, "Camera"=w87:T9, "Greyscale"=w81:bool)
                            "Greyscale" <- w81
                            n153 = call <vilib>:"IMAQdx Grab2.vi"("error in"=w94, "Wait for Next Buffer? (Yes)"=FALSE, "Image In"=w95, "Session In"=w96) -> ("error out"=w89:errorcluster, "Buffer Number Out"=w90:u32, "Image Out"=w84:T1, "Session Out"=w91:T9)  [unwired: 4 in]
                            n154 = Not A Number/Path/Refnum?(number/path/refnum=w84) -> (NaN/Path/Refnum?=w92:bool)
                            n155 = call "IMAQdx Calculate Frames per Second 1.vi"("Session In"=w91, "Buffer Number"=w90, "Minimum Display Update Interval (ms)"=w82, "Frames per Second Update Interval (ms)"=w82, "error in (no error)"=w89) -> ("Processed Frames per Second"=w88:dbl, "error out"=w85:errorcluster)  [unwired: 4 in, 5 out]
                            n156 = case shown="False" w92 {
                              tunnel: w84 -> [w102 _]
                              tunnel: [w103 _] -> w93
                              tunnel: w87 -> [_ _]
                              tunnel: w85 -> [_ _]
                              tunnel: w81 -> [w101 _]
                              frame False {
                                n157 = case shown="True" w101 {
                                tunnel: w102 -> [w104 w106]
                                tunnel: [w104 w105] -> w100
                                frame False {
                                }
                                frame True {
                                w107 = 7 items=["Red", "Green", "Blue", "Hue", "Saturation", "Luminance", "Value", "Intensity"] ("Color Plane")
                                n158 = call "IMAQ ExtractSingleColorPlane"("Color Plane"=w107, "Image Src"=w106) -> ("Image Dst Out"=w105:T1)  [unwired: 8 in, 1 out]
                                }
                                }
                                "Camera Image" <- w100
                                n159 = First Call?() -> (First Call?: T/F=w103:bool)
                              }
                              frame True {
                              }
                            }
                            n160 = Bundle By Name(cluster=w97, "error"=w85) -> (w86:T6)
                            n161 = call <vilib>:"Mean PtByPt.vi"("x"=w88, "sample length"=25) -> ("mean"=→"Frames per Second":dbl)  [unwired: 2 in, 1 out]
                            n162 = case shown="True" w93 {
                              tunnel: w87 -> [_ w98]
                              frame False {
                              }
                              frame True {
                                n163 = call "Event Generate Event.vi"("Camera Name"=w98, "Event Type"=Event_Setup_Types."Camera Loop Started") -> ()  [unwired: 10 in]
                              }
                            }
                          }
                          frame True {
                            w108 = T7 [enum."Exit"] items=["Message Dispatcher", "INI", "End Session", "Camera Process Settings", "Get Values", "Get VideoMode", "Open Settings", "Save Settings", "Set Value", "Set VideoMode", "Set WB", "Setup Camera", "Start Session", "Exit"] ("Main Queue")
                            n164 = Bundle By Name(cluster=w110, "Main Queue"=w108) -> (w109:T6)
                          }
                        }
                      }
                      frame Error {
                        w116 = T7 [enum."End Session", enum."INI", enum."Setup Camera", enum."Start Session"] items=["Message Dispatcher", "INI", "End Session", "Camera Process Settings", "Get Values", "Get VideoMode", "Open Settings", "Save Settings", "Set Value", "Set VideoMode", "Set WB", "Setup Camera", "Start Session", "Exit"] ("Main Queue")
                        # "Wait to give time for the camera to connect."
                        # "If there is an error while this loop is running we end the camera session and restart the session. Then we set the camera back up."
                        n165 = Unbundle By Name(w113) -> ("Camera"=w112:T9)
                        n166 = call "Create Camera Map Queue.vi"("Action"=enum16{"Read", "Write"}."Write", "Image in"=T1 refnum, "Camera"=w112) -> ()  [unwired: 7 in, 2 out]
                        n167 = call "Main Add to Queue.vi"("Main Queue"=w116, "Main Cluster In"=w113) -> ("Main Cluster Out"=w117:T6)  [unwired: 9 in]
                        n168 = Wait (ms)(milliseconds to wait=u32 1000) -> ()  [unwired: 1 out]
                      }
                    }
                  }
                  event User Event {
                    # "WeLook to see if this is the correct camera before we process the event. This allows us to use any camera we want an have special condition for each camera."
                    # "\"Camera Events\": are processed in this event case. These events will come from the generate camera event VI."
                    n169 = event-data() -> ("Event Type"=w122:T10, "Setpoint"=w130:i64, "Camera"=w129:string)  [unwired: 1 in]
                    n170 = local read "Camera Name 2"() -> (w120:string)
                    n171 = Equal?(x=Event_Setup_Types."Save Data", y=w122) -> (x = y?=w123:bool)
                    n172 = Equal?(x=Event_Setup_Types."Exit", y=w122) -> (x = y?=w127:bool)
                    n173 = Equal?(x=w129, y=w120) -> (x = y?=w126:bool)
                    n174 = Compound Arithmetic op=OR(w123, w127, w126) -> (w125:bool)
                    n175 = case shown="True" w125 {
                      tunnel: w121 -> [w133 w137]
                      tunnel: [w133 w138] -> w131
                      tunnel: w130 -> [_ w141]
                      tunnel: w122 -> [_ w139]
                      tunnel: w119 -> [w132 w135]
                      tunnel: [w132 w134] -> w118
                      frame False {
                      }
                      frame True {
                        n176 = case shown="\"GreyScale\"" w139 {
                          tunnel: w141 -> [_ _ _ w154 _ _ _]
                          tunnel: [w144 _ _ _ _ w165 w168] -> w140
                          tunnel: w137 -> [w143 w146 w148 w156 w162 w164 w167]
                          tunnel: [w143 w146 w148 w155 w162 w164 w167] -> w136
                          tunnel: w135 -> [w142 w145 w147 w152 w157 w163 w166]
                          tunnel: [w142 w145 w147 w149 w157 w163 w166] -> w134
                          frame Default {
                            w144 = T7 [] items=["Message Dispatcher", "INI", "End Session", "Camera Process Settings", "Get Values", "Get VideoMode", "Open Settings", "Save Settings", "Set Value", "Set VideoMode", "Set WB", "Setup Camera", "Start Session", "Exit"] ("Main Queue")
                          }
                          frame "Camera Loop Started" {
                          }
                          frame "Default" {
                          }
                          frame "GreyScale" {
                            n177 = Not Equal To 0?(x=w154) -> (x != 0?=w153:bool)
                            n178 = Bundle By Name(cluster=w156, "Greyscale"=w153) -> (w155:T6)
                            n179 = Decrement(x=w152) -> (x-1=w151:u32)
                            n180 = Decrement(x=w151) -> (x-1=w150:u32)
                            n181 = Decrement(x=w150) -> (x-1=w149:u32)
                          }
                          frame "Camera Loop Started" {
                            n182 = control-ref of="This VI"() -> (w159:refnum<vi>)
                            n183 = invoke class="VI" method="FP.Open"(reference=w159, "State"=T11."Standard") -> (reference out=w158:refnum<vi>)  [unwired: 3 in, 4 out]
                            n184 = property class="VI"(reference=w158, "FP.Behavior"=T12."Floating" ("Front Panel Window:Behavior")) -> ()  [unwired: 1 in, 2 out]
                          }
                          frame "Save Data" {
                            w165 = T7 [enum."Save Settings"] items=["Message Dispatcher", "INI", "End Session", "Camera Process Settings", "Get Values", "Get VideoMode", "Open Settings", "Save Settings", "Set Value", "Set VideoMode", "Set WB", "Setup Camera", "Start Session", "Exit"] ("Main Queue")
                          }
                          frame "Exit" {
                            w168 = T7 [enum."End Session", enum."Exit"] items=["Message Dispatcher", "INI", "End Session", "Camera Process Settings", "Get Values", "Get VideoMode", "Open Settings", "Save Settings", "Set Value", "Set VideoMode", "Set WB", "Setup Camera", "Start Session", "Exit"] ("Main Queue")
                          }
                        }
                        n185 = call "Main Add to Queue.vi"("Main Queue"=w140, "Main Cluster In"=w136) -> ("Main Cluster Out"=w138:T6)  [unwired: 9 in]
                      }
                    }
                  }
                  event "Exposure": Mouse Up {
                    w176 = T7 [enum."Set Value"] items=["Message Dispatcher", "INI", "End Session", "Camera Process Settings", "Get Values", "Get VideoMode", "Open Settings", "Save Settings", "Set Value", "Set VideoMode", "Set WB", "Setup Camera", "Start Session", "Exit"] ("Main Queue")
                    # "Camera Exposure: This is the array of states that are required to changed the exposure on the camera. This may be different for every USB camera model."
                    n186 = event-data() -> ("CtlRef"=w174:refnum<vi>)  [unwired: 1 in]
                    n187 = property class="Slide (strict)"(reference=w174) -> ("Value"=w173:i32, "Label.Text"=w171:string)  [unwired: 1 in, 2 out]
                    n188 = Build Array(w173) -> (w172:i32[])
                    n189 = Build Array(w171) -> (w170:string[])
                    n190 = call "Main Add to Queue.vi"("Main Queue"=w176, "Main Cluster In"=w177) -> ("Main Cluster Out"=w178:T6)  [unwired: 9 in]
                    n191 = Bundle By Name(cluster=w178, "Values"=w172, "Attr String"=w170) -> (w175:T6)
                  }
                  event "Contrast": Mouse Up {
                    w186 = T7 [enum."Set Value"] items=["Message Dispatcher", "INI", "End Session", "Camera Process Settings", "Get Values", "Get VideoMode", "Open Settings", "Save Settings", "Set Value", "Set VideoMode", "Set WB", "Setup Camera", "Start Session", "Exit"] ("Main Queue")
                    # "Camera Exposure: This is the array of states that are required to changed the exposure on the camera. This may be different for every USB camera model."
                    n192 = event-data() -> ("CtlRef"=w184:refnum<vi>)  [unwired: 1 in]
                    n193 = property class="Slide (strict)"(reference=w184) -> ("Label.Text"=w181:string, "Value"=w183:i32)  [unwired: 1 in, 2 out]
                    n194 = Build Array(w181) -> (w180:string[])
                    n195 = Build Array(w183) -> (w182:i32[])
                    n196 = call "Main Add to Queue.vi"("Main Queue"=w186, "Main Cluster In"=w187) -> ("Main Cluster Out"=w188:T6)  [unwired: 9 in]
                    n197 = Bundle By Name(cluster=w188, "Attr String"=w180, "Values"=w182) -> (w185:T6)
                  }
                  event "Brightness": Mouse Up {
                    w196 = T7 [enum."Set Value"] items=["Message Dispatcher", "INI", "End Session", "Camera Process Settings", "Get Values", "Get VideoMode", "Open Settings", "Save Settings", "Set Value", "Set VideoMode", "Set WB", "Setup Camera", "Start Session", "Exit"] ("Main Queue")
                    # "Bringness: When the brigness is changed it fires this event to update the brightness."
                    n198 = event-data() -> ("CtlRef"=w194:refnum<vi>)  [unwired: 1 in]
                    n199 = property class="Slide (strict)"(reference=w194) -> ("Label.Text"=w192:string, "Value"=w193:i32)  [unwired: 1 in, 2 out]
                    n200 = Build Array(w193) -> (w190:i32[])
                    n201 = Build Array(w192) -> (w191:string[])
                    n202 = call "Main Add to Queue.vi"("Main Queue"=w196, "Main Cluster In"=w197) -> ("Main Cluster Out"=w198:T6)  [unwired: 9 in]
                    n203 = Bundle By Name(cluster=w198, "Attr String"=w191, "Values"=w190) -> (w195:T6)
                  }
                  event "Save 2": Mouse Up {
                    w200 = T7 [enum."Save Settings"] items=["Message Dispatcher", "INI", "End Session", "Camera Process Settings", "Get Values", "Get VideoMode", "Open Settings", "Save Settings", "Set Value", "Set VideoMode", "Set WB", "Setup Camera", "Start Session", "Exit"] ("Main Queue")
                    # "Save Settings: When this event is fired it will send the state to save the current settings to the setup file."
                    n204 = event-data() -> ()  [unwired: 1 in, 1 out]
                    n205 = call "Main Add to Queue.vi"("Main Queue"=w200, "Main Cluster In"=w201) -> ("Main Cluster Out"=w202:T6)  [unwired: 9 in]
                  }
                  event "Sharpness": Mouse Up {
                    w210 = T7 [enum."Set Value"] items=["Message Dispatcher", "INI", "End Session", "Camera Process Settings", "Get Values", "Get VideoMode", "Open Settings", "Save Settings", "Set Value", "Set VideoMode", "Set WB", "Setup Camera", "Start Session", "Exit"] ("Main Queue")
                    # "Save Settings: When this event is fired it will send the state to save the current settings to the setup file."
                    n206 = event-data() -> ("CtlRef"=w208:refnum<vi>)  [unwired: 1 in]
                    n207 = property class="Slide (strict)"(reference=w208) -> ("Value"=w207:i32, "Label.Text"=w206:string)  [unwired: 1 in, 2 out]
                    n208 = Build Array(w207) -> (w204:i32[])
                    n209 = Build Array(w206) -> (w205:string[])
                    n210 = call "Main Add to Queue.vi"("Main Queue"=w210, "Main Cluster In"=w211) -> ("Main Cluster Out"=w212:T6)  [unwired: 9 in]
                    n211 = Bundle By Name(cluster=w212, "Values"=w204, "Attr String"=w205) -> (w209:T6)
                  }
                  event "Gamma": Mouse Up {
                    w220 = T7 [enum."Set Value"] items=["Message Dispatcher", "INI", "End Session", "Camera Process Settings", "Get Values", "Get VideoMode", "Open Settings", "Save Settings", "Set Value", "Set VideoMode", "Set WB", "Setup Camera", "Start Session", "Exit"] ("Main Queue")
                    # "Save Settings: When this event is fired it will send the state to save the current settings to the setup file."
                    n212 = event-data() -> ("CtlRef"=w218:refnum<vi>)  [unwired: 1 in]
                    n213 = property class="Slide (strict)"(reference=w218) -> ("Value"=w217:i32, "Label.Text"=w216:string)  [unwired: 1 in, 2 out]
                    n214 = Build Array(w217) -> (w214:i32[])
                    n215 = Build Array(w216) -> (w215:string[])
                    n216 = call "Main Add to Queue.vi"("Main Queue"=w220, "Main Cluster In"=w221) -> ("Main Cluster Out"=w222:T6)  [unwired: 9 in]
                    n217 = Bundle By Name(cluster=w222, "Values"=w214, "Attr String"=w215) -> (w219:T6)
                  }
                  event "Hue": Mouse Up {
                    w230 = T7 [enum."Set Value"] items=["Message Dispatcher", "INI", "End Session", "Camera Process Settings", "Get Values", "Get VideoMode", "Open Settings", "Save Settings", "Set Value", "Set VideoMode", "Set WB", "Setup Camera", "Start Session", "Exit"] ("Main Queue")
                    # "Save Settings: When this event is fired it will send the state to save the current settings to the setup file."
                    n218 = event-data() -> ("CtlRef"=w228:refnum<vi>)  [unwired: 1 in]
                    n219 = property class="Slide (strict)"(reference=w228) -> ("Value"=w227:i32, "Label.Text"=w226:string)  [unwired: 1 in, 2 out]
                    n220 = Build Array(w227) -> (w224:i32[])
                    n221 = Build Array(w226) -> (w225:string[])
                    n222 = call "Main Add to Queue.vi"("Main Queue"=w230, "Main Cluster In"=w231) -> ("Main Cluster Out"=w232:T6)  [unwired: 9 in]
                    n223 = Bundle By Name(cluster=w232, "Values"=w224, "Attr String"=w225) -> (w229:T6)
                  }
                  event "Saturation": Mouse Up {
                    w240 = T7 [enum."Set Value"] items=["Message Dispatcher", "INI", "End Session", "Camera Process Settings", "Get Values", "Get VideoMode", "Open Settings", "Save Settings", "Set Value", "Set VideoMode", "Set WB", "Setup Camera", "Start Session", "Exit"] ("Main Queue")
                    # "Save Settings: When this event is fired it will send the state to save the current settings to the setup file."
                    n224 = event-data() -> ("CtlRef"=w238:refnum<vi>)  [unwired: 1 in]
                    n225 = property class="Slide (strict)"(reference=w238) -> ("Value"=w237:i32, "Label.Text"=w236:string)  [unwired: 1 in, 2 out]
                    n226 = Build Array(w237) -> (w234:i32[])
                    n227 = Build Array(w236) -> (w235:string[])
                    n228 = call "Main Add to Queue.vi"("Main Queue"=w240, "Main Cluster In"=w241) -> ("Main Cluster Out"=w242:T6)  [unwired: 9 in]
                    n229 = Bundle By Name(cluster=w242, "Values"=w234, "Attr String"=w235) -> (w239:T6)
                  }
                  event Value Change {
                    w246 = T7 [enum."Set WB"] items=["Message Dispatcher", "INI", "End Session", "Camera Process Settings", "Get Values", "Get VideoMode", "Open Settings", "Save Settings", "Set Value", "Set VideoMode", "Set WB", "Setup Camera", "Start Session", "Exit"] ("Main Queue")
                    # "White Balance: when the whitebalance value is changed it will fire this event and cause the state to be added to the message queue."
                    n230 = event-data() -> ("NewVal"=w244:T3)  [unwired: 1 in]
                    n231 = call "Main Add to Queue.vi"("Main Queue"=w246, "Main Cluster In"=w247) -> ("Main Cluster Out"=w248:T6)  [unwired: 9 in]
                    n232 = Bundle By Name(cluster=w248, "White Balance"=w244) -> (w245:T6)
                  }
                  event "VideoMode": Value Change {
                    w250 = T7 [enum."End Session", enum."Start Session", enum."Setup Camera", enum."Get Values"] items=["Message Dispatcher", "INI", "End Session", "Camera Process Settings", "Get Values", "Get VideoMode", "Open Settings", "Save Settings", "Set Value", "Set VideoMode", "Set WB", "Setup Camera", "Start Session", "Exit"] ("Main Queue")
                    n233 = event-data() -> ("NewVal"=w251:u16)  [unwired: 1 in]
                    n234 = Bundle By Name(cluster=w254, "VideoMode"=w251) -> (w253:T6)
                    n235 = call "Main Add to Queue.vi"("Main Queue"=w250, "Main Cluster In"=w253) -> ("Main Cluster Out"=w252:T6)  [unwired: 9 in]
                  }
                  event "Close": Mouse Up {
                    n236 = event-data() -> ()  [unwired: 1 in, 1 out]
                    n237 = control-ref of="This VI"() -> (w256:refnum<vi>)
                    n238 = invoke class="VI" method="FP.Close"(reference=w256) -> ()  [unwired: 2 in, 3 out]
                  }
                }
              }
              frame "INI" {
                # "We set up all of the values to the default value. You can change these values based on the cameras that you are using as well as different envionemntal conditions that my exist in your location."
                n239 = Bundle By Name(cluster=w273, "White Balance"="White Balance", "VideoMode"="VideoMode") -> (w272:T6)
                n240 = control-ref of="Brightness"() -> (w266:refnum<vi>)
                n241 = control-ref of="Exposure"() -> (w267:refnum<vi>)
                n242 = control-ref of="Saturation"() -> (w265:refnum<vi>)
                n243 = control-ref of="Hue"() -> (w264:refnum<vi>)
                n244 = control-ref of="Gamma"() -> (w263:refnum<vi>)
                n245 = control-ref of="Contrast"() -> (w262:refnum<vi>)
                n246 = control-ref of="Sharpness"() -> (w261:refnum<vi>)
                n247 = control-ref of="Gain"() -> (w260:refnum<vi>)
                n248 = Build Array(w266, w267, w265, w264, w263, w262, w261, w260) -> (w259:refnum<vi>[])
                n249 = for {
                  tunnel: w259 -> [w277] mode=indexing
                  tunnel: [w276] -> w270 mode=indexing
                  tunnel: [w275] -> w269 mode=indexing
                  n250 = property class="Slide (strict)"(reference=w277) -> ("Label.Text"=w276:string, "Value"=w275:i32)  [unwired: 1 in, 2 out]
                }
                n251 = Bundle By Name(cluster=w272, "Controls"=w259, "Attr String"=w270, "Values"=w269) -> (w268:T6)
              }
              frame "End Session" {
                # "This state will end the camera session"
                n252 = Unbundle By Name(w284) -> ("Camera Session"=w283:T9, "error"=w279:errorcluster)
                n253 = call <vilib>:"IMAQdx Close Camera.vi"("error in"=w279, "Session In"=w283) -> ("error out"=w278:errorcluster)  [unwired: 9 in]
                n254 = call <vilib>:"Clear Errors.vi"("error in (no error)"=w278) -> ("error out"=w280:errorcluster)  [unwired: 5 in, 1 out]
                n255 = Bundle By Name(cluster=w284, "error"=w280) -> (w281:T6)
              }
              frame "Camera Process Settings" {
                w285 = T7 [enum."Set WB", enum."Set Value"] items=["Message Dispatcher", "INI", "End Session", "Camera Process Settings", "Get Values", "Get VideoMode", "Open Settings", "Save Settings", "Set Value", "Set VideoMode", "Set WB", "Setup Camera", "Start Session", "Exit"] ("Main Queue")
                # "This event finds the cameras that I am looking for and get the alias name for the camera. You can do this any way you want to. This is an easy system that is bult into LabVIEW.  I look for the camera name I am looking for and send the alias on so the camera session can be set up."
                n256 = Bundle By Name(cluster=w288, "error"=errorcluster {"status"=FALSE, "code"=0, "source"=""}, "Main Queue"=w285) -> (w286:T6)
              }
              frame "Get Values" {
                # "This step gets all the current setting in the camera if an INI file does not exist."
                n257 = Unbundle By Name(w292) -> ("Controls"=w290:refnum<vi>[], "Camera Session"=w297:T9, "Attr String"=w293:string[], "error"=w296:errorcluster)
                n258 = for {
                  tunnel: w293 -> [w303] mode=indexing
                  shift-right: [w304] -> w295
                  shift-left: w296 -> [w305]
                  shift-right: [w302] -> w294
                  shift-left: w297 -> [w306]
                  tunnel: w290 -> [w300] mode=indexing
                  n259 = call "CameraGetScaledAttrSharpness.vi"("error in (no error)"=w305, "Attr String"=w303, "IMAQdx Session"=w306) -> ("error out"=w301:errorcluster, "Scaled"=w299:dbl, "IMAQdx Session out"=w302:T9)  [unwired: 5 in, 1 out]
                  n260 = property class="Slide (strict)"(reference=w300, "Value"=w299) -> ()  [unwired: 1 in, 2 out]
                  n261 = call <vilib>:"Clear Errors.vi"("error in (no error)"=w301) -> ("error out"=w304:errorcluster)  [unwired: 5 in, 1 out]
                }
                n262 = Bundle By Name(cluster=w292, "Camera Session"=w294, "error"=w295) -> (w291:T6)
              }
              frame "Get VideoMode" {
                # "This frame sets the frame rate and picture size for the different camera models."
                n263 = Unbundle By Name(w329) -> ("Camera Session"=w331:T9, "error"=w330:errorcluster)
                n264 = call "CameraSetModeAttr.vi"("error in"=w330, "Attr String"="VideoMode", "IMAQdx Session In"=w331) -> ("error out"=w323:errorcluster, "IMAQdx Session out"=w326:T9)  [unwired: 7 in]
                n265 = property class="IMAQdx"(reference=w326, error in=w323) -> (reference out=w325:T9, error out=w324:errorcluster, "VideoMode"=w308:u32)
                n266 = property on="VideoMode" class="Ring (strict)"() -> ("Strings []"=w322:string[])  [unwired: 2 in, 2 out]
                n267 = local write "VideoMode"(w308) -> ()
                n268 = call <vilib>:"Clear Errors.vi"("error in (no error)"=w324) -> ("error out"=w315:errorcluster)  [unwired: 5 in, 1 out]
                n269 = Index Array(array=w322, index=w308) -> (element=w321:string)
                n270 = Bundle By Name(cluster=w329, "Camera Session"=w325, "error"=w315) -> (w328:T6)
                n271 = xnode "Match Regular Expression"("input string"=w321, "regular expression"="\\d++(\\.\\d{2})") -> ("whole match"=w319:string)  [unwired: 4 in, 4 out]
                n272 = Fract/Exp String To Number(string=w319, default (0 dbl)=u32 0 ("default (0 DBL)")) -> (number=w312:u32)  [unwired: 2 in, 1 out]
                n273 = Equal To 0?(x=w312) -> (x = 0?=w313:bool)
                n274 = Select(t=u32 10, s=w313, f=w312) -> (s? t:f=w309:u32)
                n275 = Reciprocal(x=w309) -> (1/x=w318:dbl)
                n276 = Multiply(x=w318, y=u32 1000) -> (x*y=w317:dbl)
                n277 = To Unsigned Long Integer(number=w317) -> (unsigned 32bit integer=w310:u32)
                n278 = Decrement(x=w310) -> (x-1=w307:u32)
              }
              frame "Open Settings" {
                # "This code opens a setup file that is used to save user preferences."
                n279 = Unbundle By Name(w455) -> ("Open And Save Controls"=w453:refnum<vi>[], "Camera"=w449:T9, "INI path"=w454:path)
                n280 = call "Attached Camera Info AE.vi"("InterfaceName"=w449) -> ("Serial Number"=w450:string)  [unwired: 10 in]
                n281 = call <vilib>:"Open Config Data.vi"("configuration file path"=w454) -> ("refnum"=w458:T18)  [unwired: 8 in, 2 out]
                n282 = for {
                  tunnel: w458 -> [w474]
                  tunnel: w450 -> [w467]
                  tunnel: w453 -> [w473] mode=indexing
                  tunnel: [w465] -> w456
                  tunnel: [w463] -> w457
                  n283 = property class="Num"(reference=w473) -> (reference out=w470:refnum<vi>, error out=w469:errorcluster, "Label.Text"=w466:string, "Value"=w461:variant)  [unwired: 1 in]
                  n284 = Variant To Flattened String(Variant=w461) -> (data string=w460:string, 1:w462:i16[])
                  n285 = call-poly <vilib>:"Read Key.vi"("section"=w467, "default value"=w460, "key"=w466, "refnum"=w474) -> ("error out"=w464:errorcluster, "value"=w471:string, "found?"=w472:bool, "refnum out"=w468:T18)  [unwired: 4 in]
                  n286 = case shown="True" w472 {
                    tunnel: w471 -> [_ w483]
                    tunnel: w470 -> [_ w488]
                    tunnel: w469 -> [_ w487]
                    tunnel: w468 -> [w481 w486]
                    tunnel: w467 -> [w480 _]
                    tunnel: w466 -> [w479 _]
                    tunnel: [w478 w486] -> w465
                    tunnel: w464 -> [w477 w485]
                    tunnel: [w476 w485] -> w463
                    tunnel: w460 -> [w475 _]
                    tunnel: w462 -> [_ w484]
                    frame False {
                      n287 = call-poly <vilib>:"Write Key.vi"("section"=w480, "error in (no error)"=w477, "value"=w475, "key"=w479, "refnum"=w481) -> ("error out"=w476:errorcluster, "refnum out"=w478:T18)  [unwired: 4 in, 1 out]
                    }
                    frame True {
                      n288 = Flattened String To Variant(6:w483, 7:w484) -> (3:w482:variant)  [unwired: 1 in, 1 out]
                      n289 = property class="Num"(reference=w488, error in=w487, "Value"=w482) -> ()  [unwired: 2 out]
                    }
                  }
                }
                n290 = call <vilib>:"Close Config Data.vi"("error in (no error)"=w457, "refnum"=w456) -> ()  [unwired: 8 in, 2 out]
                n291 = call "Stall Data Flow.vim"("value in"=w455, "milliseconds to wait"=u32 100) -> ("value out"=w452:T6)  [unwired: 1 out]
              }
              frame "Save Settings" {
                # "We save the camera setting that are important to a file so we can recall them later. The save function can be called anywhere this system is being used within the vision computer using the event fire. This can be found in frame zero of this code in the diable diagram."
                n292 = Unbundle By Name(w493) -> ("Camera"=w490:T9, "INI path"=w492:path, "Open And Save Controls"=w491:refnum<vi>[])
                n293 = call "Attached Camera Info AE.vi"("InterfaceName"=w490) -> ("Serial Number"=w489:string)  [unwired: 10 in]
                n294 = call <vilib>:"Open Config Data.vi"("configuration file path"=w492) -> ("error out"=w494:errorcluster, "refnum"=w497:T18)  [unwired: 8 in, 1 out]
                n295 = for {
                  tunnel: w491 -> [w506] mode=indexing
                  tunnel: w497 -> [w508]
                  tunnel: w489 -> [w507]
                  tunnel: [w503] -> w496
                  tunnel: [w501] -> w495
                  tunnel: w494 -> [w500]
                  n296 = property class="Num"(reference=w506, error in=w500) -> (error out=w502:errorcluster, "Label.Text"=w505:string, "Value"=w504:variant)  [unwired: 1 out]
                  n297 = Variant To Flattened String(Variant=w504) -> (data string=w499:string)  [unwired: 1 out]
                  n298 = call-poly <vilib>:"Write Key.vi"("section"=w507, "error in (no error)"=w502, "value"=w499, "key"=w505, "refnum"=w508) -> ("error out"=w501:errorcluster, "refnum out"=w503:T18)  [unwired: 4 in, 1 out]
                }
                n299 = call <vilib>:"Close Config Data.vi"("error in (no error)"=w495, "refnum"=w496) -> ()  [unwired: 8 in, 2 out]
              }
              frame "Set Value" {
                # "This frame sets the frame rate and picture size for the different camera models."
                n300 = Unbundle By Name(w511) -> ("Camera Session"=w516:T9, "Attr String"=w509:string[], "error"=w515:errorcluster, "Values"=w512:u16[])
                n301 = for {
                  tunnel: w512 -> [w518] mode=indexing
                  tunnel: w509 -> [w520] mode=indexing
                  shift-right: [w521] -> w514
                  shift-left: w515 -> [w524]
                  shift-right: [w522] -> w513
                  shift-left: w516 -> [w526]
                  n302 = call "CameraSetModeAttr.vi"("error in"=w524, "Attr String"=w520, "IMAQdx Session In"=w526) -> ("error out"=w523:errorcluster, "IMAQdx Session out"=w525:T9)  [unwired: 7 in]
                  n303 = call "CameraSetScaledAttr.vi"("error in"=w523, "Scaled"=w518, "Attr String"=w520, "IMAQdx Session in"=w525) -> ("error out"=w519:errorcluster, "IMAQdx Session"=w522:T9)  [unwired: 6 in]
                  n304 = call <vilib>:"Clear Errors.vi"("error in (no error)"=w519) -> ("error out"=w521:errorcluster)  [unwired: 5 in, 1 out]
                }
                n305 = Bundle By Name(cluster=w511, "Camera Session"=w513, "error"=w514) -> (w510:T6)
              }
              frame "Set WB" {
                w537 = 0.0 ("Color Temp (K)")
                # "Here is where you set the White Balance for the camera. We also notify the NT table so the control on the processing software and dashboard can be updated if something is changed in this software. By sending this to the NT table we keep everything syncronized."
                n306 = Unbundle By Name(w529) -> ("Camera Session"=w533:T9, "error"=w530:errorcluster, "White Balance"=w527:T3)
                n307 = call "CameraWhiteBalanceConstants.vi"() -> ("Color Temps (K)"=w536:dbl[])  [unwired: 11 in]
                n308 = Build Array (concatenate)(w536, w537, w537) -> (w535:dbl[])
                n309 = case shown="Default" w527 {
                  selector: w527 -> [w550 w559]
                  tunnel: w535 -> [w551 _]
                  tunnel: "CameraAttributes::WhiteBalance::Value" -> [w548 _]
                  tunnel: [w546 w553] -> w531
                  tunnel: w533 -> [w544 w557]
                  tunnel: "WhiteBalance" -> [w543 w556]
                  tunnel: [w542 w554] -> w532
                  tunnel: w530 -> [w541 w552]
                  frame Default {
                    n310 = Decrement(x=w550) -> (x-1=w549:T3)
                    n311 = call "CameraSetModeAttr.vi"("error in"=w541, "Attr String"=w543, "IMAQdx Session In"=w544) -> ("error out"=w540:errorcluster, "IMAQdx Session out"=w545:T9)  [unwired: 7 in]
                    n312 = Index Array(array=w551, index=w549) -> (element=w547:dbl)
                    n313 = property class="IMAQdx"(reference=w545, error in=w540, "ActiveAttribute"=w548, "ValueDBL"=w547) -> (reference out=w542:T9, error out=w546:errorcluster)
                  }
                  frame "Auto", "Hold current" {
                    n314 = Equal To 0?(x=w559) -> (x = 0?=w558:bool)
                    n315 = Select(t="Auto", s=w558, f="Manual") -> (s? t:f=w555:string)
                    n316 = call "CameraSetModeAttr.vi"("error in"=w552, "Value"=w555, "Attr String"=w556, "IMAQdx Session In"=w557) -> ("error out"=w553:errorcluster, "IMAQdx Session out"=w554:T9)  [unwired: 6 in]
                  }
                }
                n317 = Bundle By Name(cluster=w529, "Camera Session"=w532, "error"=w531) -> (w539:T6)
              }
              frame "Setup Camera" {
                # "Reg Ex to find the frame rate so we can adjust the loop speed."
                # "This state sets up the placeholder for the camera image."
                n318 = Unbundle By Name(w589) -> ("Camera"=w581:T9, "VideoMode"=w563:u16)
                n319 = call <vilib>:"IMAQdx Open Camera.vi"("error in"=errorcluster {"status"=FALSE, "code"=0, "source"=""}, "Session In"=w581) -> ("error out"=w562:errorcluster, "Session Out"=w566:T9)  [unwired: 8 in]
                n320 = call "IMAQ Create"("Border Size"=0, "Image Name"=w581) -> ("New Image"=w582:T1)  [unwired: 3 in, 1 out]
                n321 = property class="IMAQdx"(reference=w566, error in=w562, "VideoMode"=w563) -> (reference out=w565:T9, error out=w564:errorcluster)
                n322 = call <vilib>:"IMAQdx Enumerate Video Modes.vi"("Session In"=w566) -> ("error out"=w586:errorcluster, "Video Modes"=w587:T19)  [unwired: 7 in, 2 out]
                n323 = for {
                  tunnel: w587 -> [w712] mode=indexing
                  tunnel: [w711] -> w569 mode=indexing
                  n324 = Unbundle By Name(w712) -> ("Video Mode Name"=w711:string)
                }
                n325 = call <vilib>:"Clear Errors.vi"("error in (no error)"=w586) -> ()  [unwired: 5 in, 2 out]
                n326 = Bundle By Name(cluster=w589, "Camera Session"=w565, "error"=w564, "Image In"=w582) -> (w585:T6)
                n327 = property on="VideoMode" class="Ring (strict)"("Strings []"=w569, "Value"=w563) -> ()  [unwired: 2 in, 2 out]
                n328 = case shown="No Error" w564 {
                  tunnel: w585 -> [w707 w710]
                  tunnel: [w707 w709] -> w584
                  frame No Error {
                  }
                  frame Error {
                    w708 = T7 [] items=["Message Dispatcher", "INI", "End Session", "Camera Process Settings", "Get Values", "Get VideoMode", "Open Settings", "Save Settings", "Set Value", "Set VideoMode", "Set WB", "Setup Camera", "Start Session", "Exit"] ("Main Queue")
                    # "Clear the queue"
                    n329 = Bundle By Name(cluster=w710, "Main Queue"=w708) -> (w709:T6)
                  }
                }
                n330 = Index Array(array=w569, index=w563) -> (element=w580:string)
                n331 = xnode "Match Regular Expression"("input string"=w580, "regular expression"="\\d++(\\.\\d{2})") -> ("whole match"=w578:string)  [unwired: 4 in, 4 out]
                n332 = Fract/Exp String To Number(string=w578, default (0 dbl)=u32 0 ("default (0 DBL)")) -> (number=w572:u32)  [unwired: 2 in, 1 out]
                n333 = Equal To 0?(x=w572) -> (x = 0?=w573:bool)
                n334 = Select(t=u32 10, s=w573, f=w572) -> (s? t:f=w570:u32)
                n335 = Reciprocal(x=w570) -> (1/x=w577:dbl)
                n336 = Multiply(x=w577, y=u32 1000) -> (x*y=w576:dbl)
                n337 = To Unsigned Long Integer(number=w576) -> (unsigned 32bit integer=w568:u32)
                n338 = Decrement(x=w568) -> (x-1=w567:u32)
              }
              frame "Start Session" {
                w716 = u32 3 items=["Get Oldest"=0, "Fail"=2, "Get Newest"=3] ("OverwriteMode")
                # "This state starts the camera session and passes it to the rest of the code so it can be used. We also get the picture size."
                n339 = Unbundle By Name(w727) -> ("Camera Session"=w713:T9, "error"=w718:errorcluster, "INI File Found"=w714:bool)
                n340 = property class="IMAQdx"(reference=w713, error in=w718, "OverwriteMode"=w716) -> (reference out=w719:T9, error out=w717:errorcluster)
                n341 = call <vilib>:"IMAQdx Configure Grab.vi"("error in"=w717, "Session In"=w719) -> ("error out"=w725:errorcluster, "Session Out"=w723:T9)  [unwired: 8 in]
                n342 = property class="IMAQdx"(reference=w723, error in=w725) -> (error out=w726:errorcluster, "Height"=→"Height 2":u32, "Width"=→"Width 2":u32)  [unwired: 1 out]
                n343 = Bundle By Name(cluster=w727, "Camera Session"=w723, "error"=w726) -> (w722:T6)
                n344 = First Call?() -> (First Call?: T/F=w720:bool)
                n345 = And(x=w720, y=w714) -> (x .and. y?=w715:bool)
                n346 = case shown="False" w715 {
                  tunnel: w722 -> [w730 w733]
                  tunnel: [w730 w732] -> w721
                  frame False {
                  }
                  frame True {
                    w731 = T7 [enum."Camera Process Settings"] items=["Message Dispatcher", "INI", "End Session", "Camera Process Settings", "Get Values", "Get VideoMode", "Open Settings", "Save Settings", "Set Value", "Set VideoMode", "Set WB", "Setup Camera", "Start Session", "Exit"] ("Main Queue")
                    n347 = call "Main Add to Queue.vi"("Main Queue"=w731, "Main Cluster In"=w733) -> ("Main Cluster Out"=w732:T6)  [unwired: 9 in]
                  }
                }
              }
              frame "Exit" {
                # "The end frame is where we shut this software down when we want to exit the program."
              }
            }
          }
        }
      }
    }
  }
